vi "Label Image.vi"(6 "Edges":T1[](array[typedef]), 8 "Line":T2, 9 "Annotate":bool=TRUE, 10 "Results":T4 {"Score" format="%#_3g"; "Pixels"."Box"."Bottom" format="%#_3g"; "Pixels"."Box"."Right" format="%#_3g"; "Pixels"."Box"."Top" format="%#_3g"; "Pixels"."Box"."Left" format="%#_3g"; "Normalized"."Box"."Bottom" format="%#_3g"; "Normalized"."Box"."Right" format="%#_3g"; "Normalized"."Box"."Top" format="%#_3g"; "Normalized"."Box"."Left" format="%#_3g"; "Distance (ft)" format="%#_3g"}, 11 "Image":T3) -> (3 "Image Out":T3)   [LabVIEW 2017, in "VisionSystem.lvlib"]
doc: "Draw text values near or on the particle and draws a square around the target stripes.."
uses:
  VisionSystem.lvlib
  Cluster_Results.ctl
  Cluster_Targeting Data.ctl
  Cluster_SGL Point.ctl
  Cluster_UI DBL Box.ctl
  <vilib>/vision/Image Controls.llb/IMAQ Image.ctl
  Cluster_Line.ctl
  Cluster_I32 Point.ctl
  Cluster_I32 Box.ctl
panel:
  out "Oval":errorcluster
  out "Line":errorcluster
  out "Rect":errorcluster
  out "tesxt":errorcluster
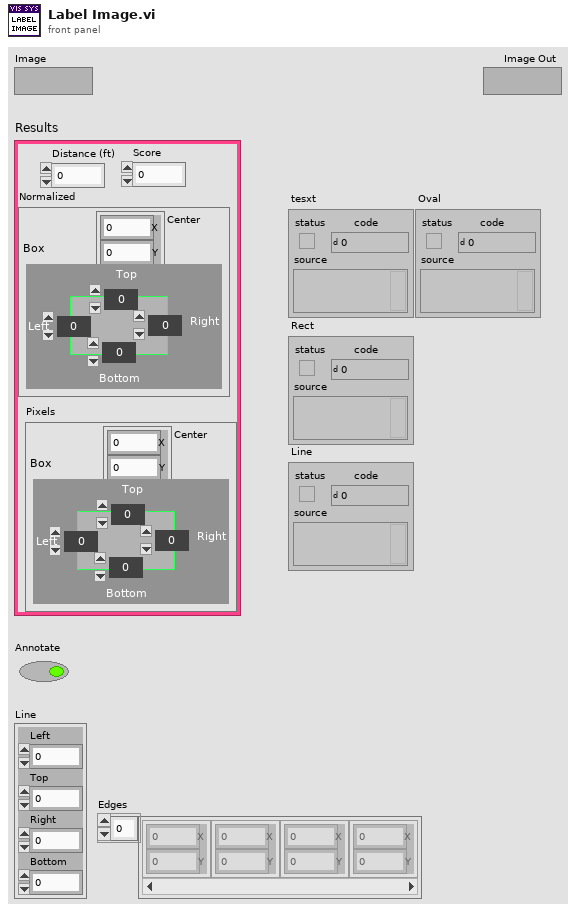
[diagram p1: front panel]
types:
  T1 = typedef "VisionSystem.lvlib/Cluster_SGL Point.ctl" = cluster{"X":sgl, "Y":sgl}
  T2 = typedef "VisionSystem.lvlib/Cluster_Line.ctl" = cluster{"Left":dbl, "Top":dbl, "Right":dbl, "Bottom":dbl}
  T3 = typedef "IMAQ Image.ctl" = refnum<image>
  T4 = typedef "VisionSystem.lvlib/Cluster_Results.ctl" = cluster{"Distance (ft)":dbl, "Score":dbl, "Normalized":T5, "Pixels":T5}
  T5 = typedef "VisionSystem.lvlib/Cluster_Targeting Data.ctl" = cluster{"Center":T1, "Box":T6}
  T6 = typedef "VisionSystem.lvlib/Cluster_UI DBL Box.ctl" = cluster{"Left":dbl, "Top":dbl, "Right":dbl, "Bottom":dbl}
  T7 = cluster{"Desired Font (Application)":enum16{"User-specified Font", "Application Font", "System Font", "Dialog Font"}, "[User-specified Font]":cluster{"Font Name":string, "Size":i16, "Strikeout?":bool, "Italic?":bool, "Underline?":bool, "Outline?":bool, "Shadow?":bool, "Bold?":bool, "Rotation Angle":dbl}, "Horizontal Alignment":i16, "Vertical Alignment":i16}
  T8 = cluster{"Left":i32, "Top":i32, "Right":i32, "Bottom":i32}
  T9 = typedef "VisionSystem.lvlib/Cluster_I32 Box.ctl" = cluster{"Left":i32, "Top":i32, "Right":i32, "Bottom":i32}
  T10 = typedef "VisionSystem.lvlib/Cluster_I32 Point.ctl" = cluster{"X":i32, "Y":i32}
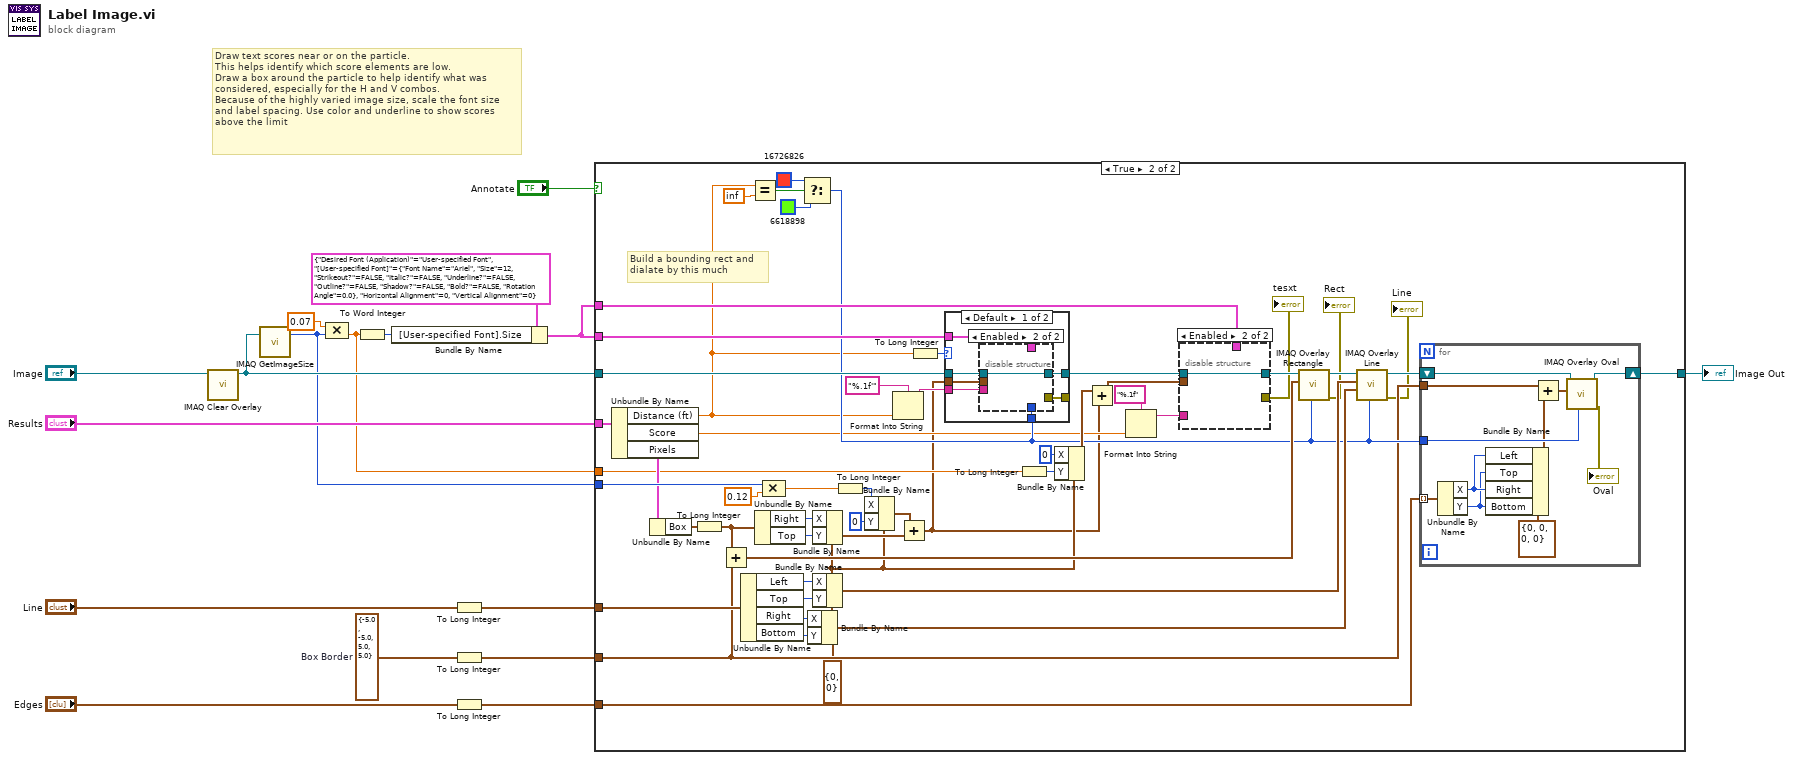
[diagram p0: block diagram]
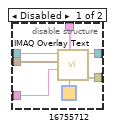
[diagram p3: hidden frame]
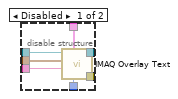
[diagram p4: hidden frame]
diagram:
  w9 = cluster{dbl, dbl, dbl, dbl} {-5.0, -5.0, 5.0, 5.0}  # Box Border
  # "Draw text scores near or on the particle.\nThis helps identify which score elements are low.\nDraw a box around the particle to help identify what was\nconsidered, especially for the H and V combos.\nBecause of the highly varied image size, scale the font size\nand label spacing. Use color and underline to show scores\nabove the limit"
  n1 = call "IMAQ Clear Overlay"("Image"="Image") -> ("Image Out"=w12:T3)  [unwired: 2 in, 8 out]
  n2 = call "IMAQ GetImageSize"("Image"=w12) -> ("Y Resolution"=w11:i32)  [unwired: 3 in, 2 out]
  n3 = Compound Arithmetic op=MULTIPLY(0.07, w11) -> (w7:dbl)
  n4 = To Word Integer(number=w7) -> (16bit integer=w1:i16)
  n5 = Bundle By Name(cluster=T7 {"Desired Font (Application)"=enum."User-specified Font", "[User-specified Font]"={"Font Name"="Ariel", "Size"=12, "Strikeout?"=FALSE, "Italic?"=FALSE, "Underline?"=FALSE, "Outline?"=FALSE, "Shadow?"=FALSE, "Bold?"=FALSE, "Rotation Angle"=0.0}, "Horizontal Alignment"=0, "Vertical Alignment"=0} ("Font, Size & Style"), "[User-specified Font].Size"=w1) -> (w8:T7)
  n6 = To Long Integer(number="Line") -> (32bit integer=w4:T8)
  n7 = To Long Integer(number=w9) -> (32bit integer=w2:cluster{i32, i32, i32, i32})
  n8 = To Long Integer(number="Edges") -> (32bit integer=w3:cluster{"X":i32, "Y":i32}[])
  n9 = case shown="True" "Annotate" {
    tunnel: [w18 w35] -> w17
    tunnel: "Results" -> [_ w71]
    tunnel: w12 -> [w18 w70]
    tunnel: w8 -> [_ w60]
    tunnel: w11 -> [_ w69]
    tunnel: w2 -> [_ w31]
    tunnel: w8 -> [_ w55]
    tunnel: w7 -> [_ w49]
    tunnel: w4 -> [_ w44]
    tunnel: w3 -> [_ w34]
    frame False {
    }
    frame True {
      w26 = T10 {"X"=0, "Y"=0} ("Location (Pixel)")
      # "Build a bounding rect and\ndialate by this much"
      n10 = Unbundle By Name(w71) -> ("Distance (ft)"=w22:dbl, "Score"=w25:dbl, "Pixels"=w58:T5)
      n11 = Unbundle By Name(w58) -> ("Box"=w59:T6)
      n12 = To Long Integer(number=w59) -> (32bit integer=w30:T8)
      n13 = Add(x=w30, y=w31) -> (x+y=w66:cluster{i32, i32, i32, i32})
      n14 = Unbundle By Name(w44) -> ("Left"=w43:i32, "Top"=w42:i32, "Right"=w41:i32, "Bottom"=w40:i32)
      n15 = Equal?(x=w22, y=inf) -> (x = y?=w46:bool)
      n16 = Unbundle By Name(w30) -> ("Right"=w68:i32, "Top"=w23:i32)
      n17 = Compound Arithmetic op=MULTIPLY(w69, 0.12) -> (w63:dbl)
      n18 = Select(t=u32 16726826 ("Color"), s=w46, f=u32 6618898 ("Color")) -> (s? t:f=w33:u32)
      n19 = Bundle By Name(cluster=w26, "X"=w41, "Y"=w40) -> (w37:T10)
      n20 = Bundle By Name(cluster=w26, "X"=w68, "Y"=w23) -> (w67:T10)
      n21 = Bundle By Name(cluster=w26, "X"=w43, "Y"=w42) -> (w38:T10)
      n22 = To Long Integer(number=w63) -> (32bit integer=w29:i32)
      n23 = Bundle By Name(cluster=w26, "X"=w29, "Y"=0) -> (w65:T10)
      n24 = Format Into String(format string="%.1f'", w22) -> (resulting string=w61:string)  [unwired: 2 in, 1 out]
      n25 = Add(x=w65, y=w67) -> (x+y=w24:T10)
      n26 = To Long Integer(number=w22) -> (32bit integer=w27:i32)
      n27 = case shown="Default" w27 {
        tunnel: w70 -> [w86 w95]
        tunnel: w61 -> [w85 _]
        tunnel: w60 -> [w84 _]
        tunnel: [w83 w95] -> w57
        tunnel: w24 -> [w82 _]
        tunnel: w33 -> [w81 _]
        tunnel: [w80 _] -> _
        frame Default {
          n28 = disable-structure shown="Enabled" {
            disable-tunnel: w86 -> [w93 w94]
            disable-tunnel: w85 -> [w92 _]
            disable-tunnel: w84 -> [w91 _]
            disable-tunnel: [w90 w94] -> w83
            disable-tunnel: w82 -> [w89 _]
            disable-tunnel: w81 -> [w88 _]
            disable-tunnel: [w87 _] -> w80
            frame Disabled {
              n29 = call "IMAQ Overlay Text"("Text Color (black)"=w88, "Font, Size & Style"=w91, "String"=w92, "Origin"=w89, "Image"=w93) -> ("error out"=w87:errorcluster, "Image Out"=w90:T3)  [unwired: 5 in]
            }
            frame Enabled {
            }
          }
        }
        frame 0 {
        }
      }
      n30 = To Long Integer(number=w49) -> (32bit integer=w28:i32)
      n31 = Bundle By Name(cluster=w26, "X"=0, "Y"=w28) -> (w52:T10)
      n32 = Add(x=w52, y=w24) -> (x+y=w50:T10)
      n33 = Format Into String(format string="%.1f", w25) -> (resulting string=w53:string)  [unwired: 2 in, 1 out]
      n34 = disable-structure shown="Enabled" {
        disable-tunnel: w57 -> [w78 w79]
        disable-tunnel: [w77 w79] -> w56
        disable-tunnel: w55 -> [w76 _]
        disable-tunnel: w53 -> [w74 _]
        disable-tunnel: w50 -> [w73 _]
        disable-tunnel: [w72 _] -> w21
        frame Disabled {
          n35 = call "IMAQ Overlay Text"("Text Color (black)"=u32 16755712 ("Color"), "Font, Size & Style"=w76, "String"=w74, "Origin"=w73, "Image"=w78) -> ("error out"=w72:errorcluster, "Image Out"=w77:T3)  [unwired: 5 in]
        }
        frame Enabled {
        }
      }
      "tesxt" <- w21
      n36 = call "IMAQ Overlay Rectangle"("Color"=w33, "Rectangle"=w66, "Image"=w56) -> ("error out"=→"Rect":errorcluster, "Image Out"=w39:T3)  [unwired: 7 in]
      n37 = call "IMAQ Overlay Line"("Color"=w33, "End Point"=w37, "Start Point"=w38, "Image"=w39) -> ("error out"=→"Line":errorcluster, "Image Out"=w36:T3)  [unwired: 6 in]
      n38 = for {
        shift-right: [w105] -> w35
        shift-left: w36 -> [w106]
        tunnel: w33 -> [w104]
        tunnel: w34 -> [w102] mode=indexing
        tunnel: w31 -> [w98]
        n39 = Unbundle By Name(w102) -> ("X"=w101:i32, "Y"=w100:i32)
        n40 = Bundle By Name(cluster=T9 {"Left"=0, "Top"=0, "Right"=0, "Bottom"=0} ("Bounding Rectangle"), "Left"=w101, "Top"=w100, "Right"=w101, "Bottom"=w100) -> (w99:T9)
        n41 = Add(x=w98, y=w99) -> (x+y=w103:T9)
        n42 = call "IMAQ Overlay Oval"("Color"=w104, "Bounding Rectangle"=w103, "Image"=w106) -> ("error out"=→"Oval":errorcluster, "Image Out"=w105:T3)  [unwired: 7 in]
      }
    }
  }
  "Image Out" <- w17
